vi "CurrentSet.vi"(8 "error in (no error)":errorcluster, 10 "Current":T1, 11 "Cluster":T3) -> (0 "error out":errorcluster, 3 "output cluster":T2)   [LabVIEW 2020, in "YP PowerControl.lvlib"]
uses:
  YP PowerControl.lvlib
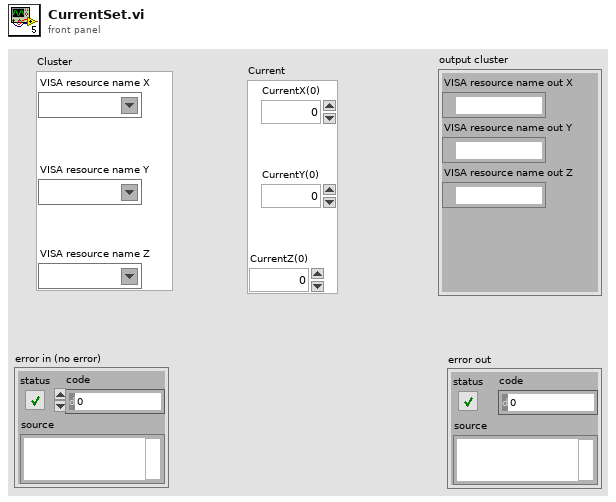
[diagram p1: front panel]
types:
  T1 = cluster{"CurrentX(0)":dbl, "CurrentY(0)":dbl, "CurrentZ(0) ":dbl}
  T2 = cluster{"VISA resource name out X":refnum<visa-resource-name>, "VISA resource name out Y":refnum<visa-resource-name>, "VISA resource name out Z":refnum<visa-resource-name>}
  T3 = cluster{"VISA resource name X":refnum<visa-resource-name>, "VISA resource name Y":refnum<visa-resource-name>, "VISA resource name Z":refnum<visa-resource-name>}
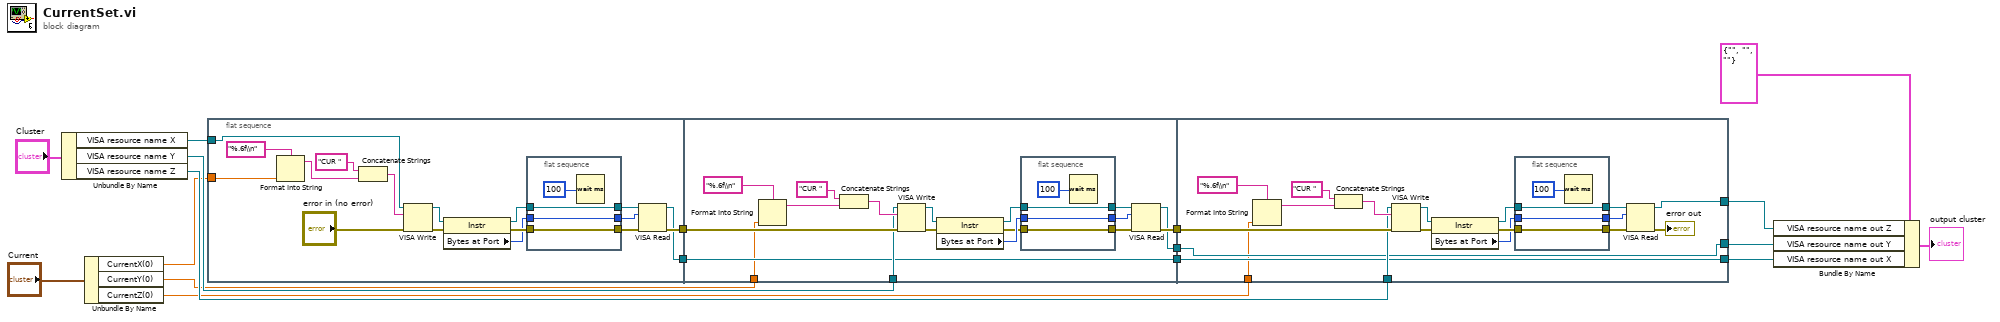
[diagram p0: block diagram]
diagram:
  n1 = Unbundle By Name("Cluster") -> ("VISA resource name X"=w15:refnum<visa-resource-name>, "VISA resource name Y"=w14:refnum<visa-resource-name>, "VISA resource name Z"=w13:refnum<visa-resource-name>)
  n2 = Unbundle By Name("Current") -> ("CurrentX(0)"=w3:dbl, "CurrentY(0)"=w2:dbl, "CurrentZ(0)"=w1:dbl)
  n3 = flat-sequence {
    tunnel: [w23] -> w18
    tunnel: w15 -> [w21]
    tunnel: [w20] -> w12
    tunnel: w3 -> [w19]
    tunnel: w18 -> [w45]
    tunnel: [w44] -> w17
    tunnel: w14 -> [w43]
    tunnel: w12 -> [w42]
    tunnel: [w42] -> w11
    tunnel: [w41] -> w10
    tunnel: w2 -> [w40]
    tunnel: w17 -> [w67]
    tunnel: w13 -> [w66]
    tunnel: w11 -> [w63]
    tunnel: [w65] -> w8
    tunnel: w10 -> [w65]
    tunnel: [w64] -> w9
    tunnel: [w63] -> w7
    tunnel: w1 -> [w62]
    frame #0 {
      n4 = Format Into String(format string="%.6f\\n", w19) -> (resulting string=w29:string)  [unwired: 2 in, 1 out]
      n5 = Concatenate Strings("CUR " ("string"), w29) -> (w24:string)
      n6 = VISA Write(VISA resource name=w21, write buffer=w24, error in (no error)="error in (no error)") -> (VISA resource name out=w26:refnum<visa-resource-name>, error out=w25:errorcluster)  [unwired: 1 out]
      n7 = property class="Instr"(reference=w26, error in=w25) -> (reference out=w32:refnum<visa-resource-name>, error out=w34:errorcluster, "Bytes at Port"=w30:u32)
      n8 = flat-sequence {
        tunnel: w32 -> [w39]
        tunnel: [w39] -> w33
        tunnel: [w38] -> w35
        tunnel: w34 -> [w38]
        tunnel: [w37] -> w31
        tunnel: w30 -> [w37]
        frame #0 {
          n9 = Wait (ms)(milliseconds to wait=u32 100) -> ()  [unwired: 1 out]
        }
      }
      n10 = VISA Read(VISA resource name=w33, byte count=w31, error in (no error)=w35) -> (VISA resource name out=w20:refnum<visa-resource-name>, error out=w23:errorcluster)  [unwired: 2 out]
    }
    frame #1 {
      n11 = Format Into String(format string="%.6f\\n", w40) -> (resulting string=w52:string)  [unwired: 2 in, 1 out]
      n12 = Concatenate Strings("CUR " ("string"), w52) -> (w57:string)
      n13 = VISA Write(VISA resource name=w43, write buffer=w57, error in (no error)=w45) -> (VISA resource name out=w55:refnum<visa-resource-name>, error out=w56:errorcluster)  [unwired: 1 out]
      n14 = property class="Instr"(reference=w55, error in=w56) -> (reference out=w49:refnum<visa-resource-name>, error out=w47:errorcluster, "Bytes at Port"=w51:u32)
      n15 = flat-sequence {
        tunnel: w49 -> [w61]
        tunnel: [w61] -> w48
        tunnel: [w60] -> w46
        tunnel: w47 -> [w60]
        tunnel: [w59] -> w50
        tunnel: w51 -> [w59]
        frame #0 {
          n16 = Wait (ms)(milliseconds to wait=u32 100) -> ()  [unwired: 1 out]
        }
      }
      n17 = VISA Read(VISA resource name=w48, byte count=w50, error in (no error)=w46) -> (VISA resource name out=w41:refnum<visa-resource-name>, error out=w44:errorcluster)  [unwired: 2 out]
    }
    frame #2 {
      n18 = Format Into String(format string="%.6f\\n", w62) -> (resulting string=w74:string)  [unwired: 2 in, 1 out]
      n19 = Concatenate Strings("CUR " ("string"), w74) -> (w69:string)
      n20 = VISA Write(VISA resource name=w66, write buffer=w69, error in (no error)=w67) -> (VISA resource name out=w71:refnum<visa-resource-name>, error out=w70:errorcluster)  [unwired: 1 out]
      n21 = property class="Instr"(reference=w71, error in=w70) -> (reference out=w77:refnum<visa-resource-name>, error out=w79:errorcluster, "Bytes at Port"=w75:u32)
      n22 = flat-sequence {
        tunnel: w77 -> [w84]
        tunnel: [w84] -> w78
        tunnel: [w83] -> w80
        tunnel: w79 -> [w83]
        tunnel: [w82] -> w76
        tunnel: w75 -> [w82]
        frame #0 {
          n23 = Wait (ms)(milliseconds to wait=u32 100) -> ()  [unwired: 1 out]
        }
      }
      n24 = VISA Read(VISA resource name=w78, byte count=w76, error in (no error)=w80) -> (VISA resource name out=w64:refnum<visa-resource-name>, error out=→"error out":errorcluster)  [unwired: 2 out]
    }
  }
  n25 = Bundle By Name(cluster=T2 {"VISA resource name out X"="", "VISA resource name out Y"="", "VISA resource name out Z"=""} ("Cluster 2"), "VISA resource name out Z"=w9, "VISA resource name out Y"=w8, "VISA resource name out X"=w7) -> (→"output cluster":T2)
